vi "Query with no type.vi"(8 "error in (no error)":errorcluster, 9 "Type":variant, 10 "Query string":string, 11 "sqlite3 in":refnum<class "sqlite3.lvclass">) -> (0 "error out":errorcluster, 2 "Variant":variant, 3 "sqlite3 out":refnum<class "sqlite3.lvclass">)   [LabVIEW 2020, in "sqlite3.lvlib" / "sqlite3.lvclass"]
uses:
  sqlite3.lvclass
  sqlite3.lvclass/sqlite3.ctl
  2bf0807a-0464-431b-84cd-0c2c6942a772.vi
  sqlite/VIs/open v2.vi
  sqlite/VIs/close v2.vi
  sqlite/VIs/prepare v2.vi
  sqlite/VIs/step.vi
  sqlite/VIs/column count.vi
  db layer/compound/Resolve Result Type.vi
  2bf0807a-0464-431b-84cd-0c2c6942a772.vi/2af19fa9-f629-455c-b9d4-1bb5c118d383.vi
  sqlite/VIs/finalize.vi
  sqlite/subvi/Error Converter (ErrCode or Status).vi
  sqlite/VIs/column type.vi
  sqlite/VIs/column bytes.vi
  sqlite/VIs/column blob.vi
  db layer/utilities/MoveBlock.vi
  sqlite/VIs/errstr.vi
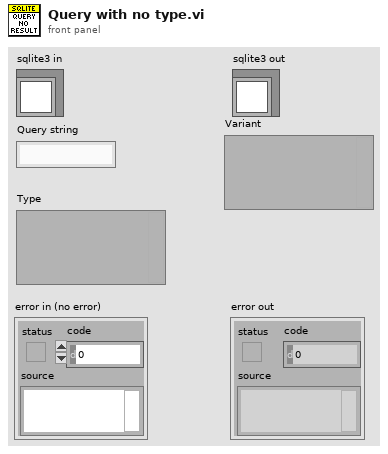
[diagram p1: front panel]
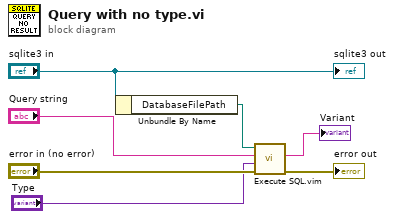
[diagram p0: block diagram]
diagram:
  n1 = Unbundle By Name("sqlite3 in") -> ("DatabaseFilePath"=w2:path)
  n2 = call "Execute SQL.vim"("error in (no error)"="error in (no error)", "desired return type(none)"="Type", "sql (string)"="Query string", "database in"=w2) -> ("error out"=→"error out":errorcluster, "Query Result"=→"Variant":string)  [unwired: 6 in]
  "sqlite3 out" <- "sqlite3 in"
